vi "Hydrolysis_stop.vi"() -> ()   [LabVIEW 2021]
panel:
  out "Hydrolysis_stop":bool
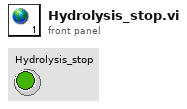
[diagram p1: front panel]
diagram:
